vi "Configure Measurement (Frequency-Power).vi"(0 "VISA resource name":refnum<visa-resource-name>, 1 "Sample Count (201)":i32=201 format="%^#_9g", 5 "Maximum Input Level (0 dBm)":dbl format="%^#_9g", 7 "Measurement Mode (0: Analyzer)":u16(ring) items=["Analyzer", "Tester"], 9 "Frequency Resolution (2: Wide)":u16(ring)=2 items=["Narrow", "Middle", "Wide"], 11 "error in (no error)":errorcluster, 12 "Sample Delay (0 s)":dbl format="%^#_9g") -> (4 "VISA resource name out":refnum<visa-resource-name>, 15 "error out":errorcluster)   [LabVIEW 2011, in "Agilent E5052X.lvlib"]
doc: "Configures the instrument to take Frequency/Power measurements.\n\n<b>Note: </b> \n\n\"Configure Measurement Characteristics(Freq-Power)\" VI must be called before calling this VI."
uses:
  Agilent E5052X.lvlib
panel:
  # "Sample Settings"
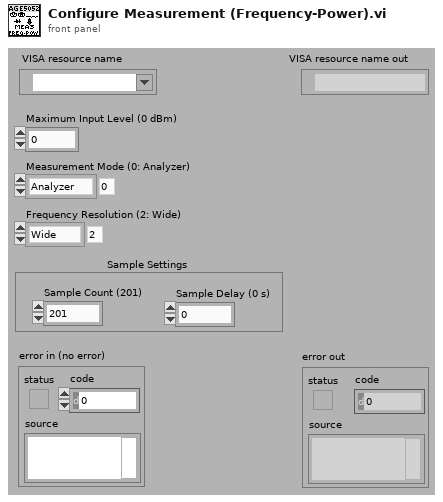
[diagram p1: front panel]
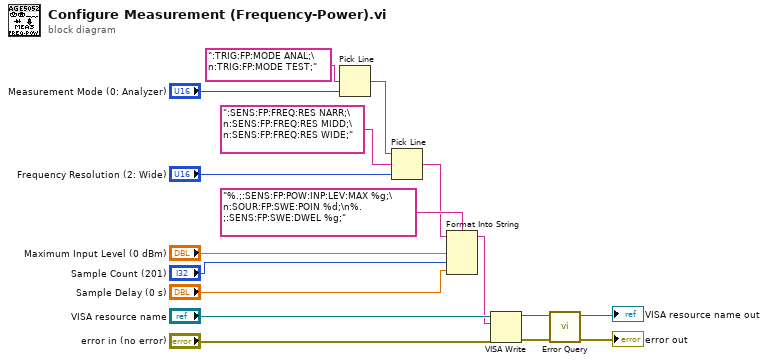
[diagram p0: block diagram]
diagram:
  n1 = Pick Line(multi-line string=":TRIG:FP:MODE ANAL;\n:TRIG:FP:MODE TEST;", line index="Measurement Mode (0: Analyzer)") -> (output string=w3:string)  [unwired: 1 in]
  n2 = Pick Line(string ("")=w3, multi-line string=":SENS:FP:FREQ:RES NARR;\n:SENS:FP:FREQ:RES MIDD;\n:SENS:FP:FREQ:RES WIDE;", line index="Frequency Resolution (2: Wide)") -> (output string=w2:string)
  n3 = Format Into String(format string="%.;:SENS:FP:POW:INP:LEV:MAX %g;\n:SOUR:FP:SWE:POIN %d;\n%.;:SENS:FP:SWE:DWEL %g;", initial string=w2, "Maximum Input Level (0 dBm)", "Sample Count (201)", "Sample Delay (0 s)") -> (resulting string=w1:string)  [unwired: 1 in, 1 out]
  n4 = VISA Write(VISA resource name="VISA resource name", write buffer=w1, error in (no error)="error in (no error)") -> (VISA resource name out=w11:refnum<visa-resource-name>, error out=w10:errorcluster)  [unwired: 1 out]
  n5 = call "Error Query.vi"("error in (no error)"=w10, "VISA resource name"=w11) -> ("error out"=→"error out":errorcluster, "VISA resource name out"=→"VISA resource name out":refnum<visa-resource-name>)  [unwired: 6 in, 2 out]
